vi "Drive.vi"   [LabVIEW 2012]
uses:
  StateMachineType.ctl
  <vilib>/Rock Robotics/WPI/RobotDrive/WPI_RobotDriveGetSetRefNum.vi
  Robot Global Data.vi
types:
  T1 = typedef "StateMachineType.ctl" = enum16{"Init", "Idle", "Start", "Do", "Stop"}
  T2 = typedef "WPI_RobotDriveDevRef.ctl" = cluster{"DevStatus":errorcluster, "Motors[]":T3[], "Square Inputs":bool, "Max Output":dbl, "Isochronous":bool}
  T3 = typedef "WPI_MotorControlDeviceRef.ctl" = cluster{"DeviceStatus":errorcluster, "Type":enum16{"PWM", "CAN"}, "PWM":cluster{"Digital Module":T4, "PWM Channel":T5, "DeadBand":T6}, "CAN":cluster{"Device Number":u8, "Control Mode":T7, "Semaphore":T8, "Max Vout":dbl}, "Invert":bool, "TransformRef":T9, "InvTransformRef":T9}
  T4 = typedef "FPGA_TypedefDigitalModule.ctl" = enum16{"Digital Module 1", "Digital Module 2"}
  T5 = typedef "FPGA_DIOPWMChannel.ctl" = enum8{"PWM 1", "PWM 2", "PWM 3", "PWM 4", "PWM 5", "PWM 6", "PWM 7", "PWM 8", "PWM 9", "PWM 10", "Invalid"}
  T6 = typedef "WPI_PWMDeadband.ctl" = cluster{"Name":string, "maxPositivePwm":i32, "minPositivePwm":i32, "centerPwm":i32, "maxNegativePwm":i32, "minNegativePwm":i32, "angularRange":u16}
  T7 = typedef "WPI_CANJaguar_ControlMode.ctl" = enum8{"Percent VBus", "Current", "Speed", "Position", "Voltage"}
  T8 = typedef "Semaphore RefNum" = refnum<k1>
  T9 = typedef "WPI_PWMTransform_ConPane.ctl" = refnum<vi>
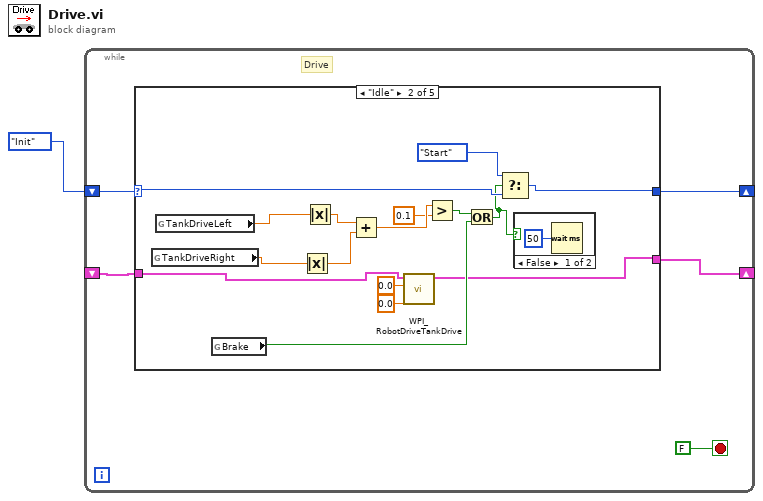
[diagram p0: block diagram]
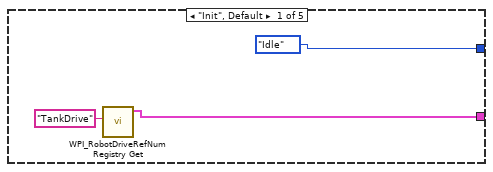
[diagram p2: hidden frame]
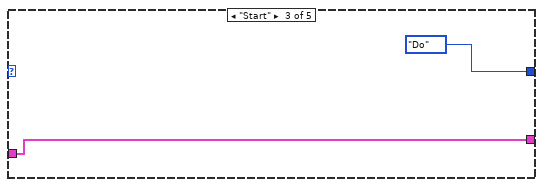
[diagram p4: hidden frame]
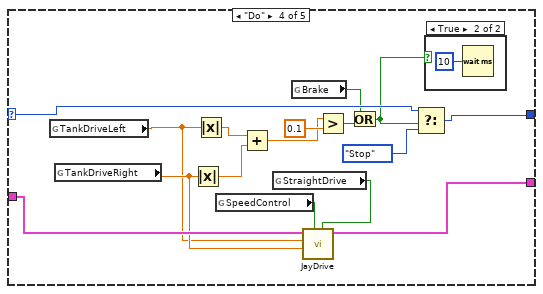
[diagram p5: hidden frame]
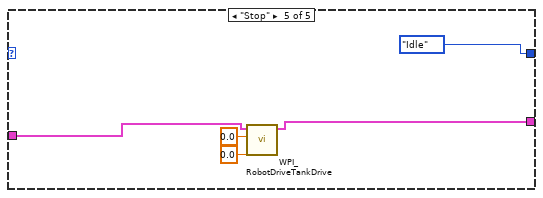
[diagram p7: hidden frame]
diagram:
  n1 = while {
    shift-right: [w4] -> _
    shift-left: StateMachineType."Init" -> [w5]
    shift-right: [w3] -> _
    shift-left: _ -> [w2]
    stop <- FALSE stop-if-true
    # "Drive"
    n2 = case shown="\"Idle\"" w5 {
      selector: w5 -> [_ w20 _ w35 _]
      tunnel: [StateMachineType."Idle" ("Enum") w19 StateMachineType."Do" ("Enum") w36 StateMachineType."Idle" ("Enum")] -> w4
      tunnel: [w7 w10 w28 w37 w48] -> w3
      tunnel: w2 -> [_ w11 w28 w38 w47]
      frame "Init", Default {
        n3 = call <vilib>:"WPI_RobotDriveRefNum Registry Get.vi"("refnum name"="TankDrive") -> ("RobotDriveDevRef"=w7:T2)  [unwired: 9 in, 1 out]
      }
      frame "Idle" {
        n4 = global read "Robot Global Data.vi" "TankDriveRight"() -> (w25:dbl)
        n5 = global read "Robot Global Data.vi" "TankDriveLeft"() -> (w17:dbl)
        n6 = global read "Robot Global Data.vi" "Brake"() -> (w15:bool)
        n7 = Absolute Value(x=w25) -> (abs(x)=w23:dbl)
        n8 = Absolute Value(x=w17) -> (abs(x)=w24:dbl)
        n9 = Add(x=w24, y=w23) -> (x+y=w22:dbl)
        n10 = call <vilib>:"WPI_RobotDriveTankDrive.vi"("Right axis value"=0.0, "Left axis value"=0.0, "RobotDriveDevRef"=w11) -> ("RobotDriveDevRef"=w10:T2)  [unwired: 6 in, 2 out]
        n11 = Greater?(x=w22, y=0.1) -> (0:w16:bool)
        n12 = Or(x=w16, y=w15) -> (x .or. y?=w14:bool)
        n13 = Select(t=StateMachineType."Start" ("Enum"), s=w14, f=w20) -> (s? t:f=w19:T1)
        n14 = case shown="False" w14 {
          frame False {
            n15 = Wait (ms)(milliseconds to wait=u32 50) -> ()  [unwired: 1 out]
          }
          frame True {
          }
        }
      }
      frame "Start" {
      }
      frame "Do" {
        n16 = global read "Robot Global Data.vi" "TankDriveLeft"() -> (w33:dbl)
        n17 = global read "Robot Global Data.vi" "TankDriveRight"() -> (w34:dbl)
        n18 = Absolute Value(x=w34) -> (abs(x)=w40:dbl)
        n19 = Absolute Value(x=w33) -> (abs(x)=w41:dbl)
        n20 = global read "Robot Global Data.vi" "SpeedControl"() -> (w39:bool)
        n21 = Add(x=w41, y=w40) -> (x+y=w43:dbl)
        n22 = global read "Robot Global Data.vi" "StraightDrive"() -> (w32:bool)
        n23 = global read "Robot Global Data.vi" "Brake"() -> (w30:bool)
        n24 = call "JayDrive.vi"("StraightDrive"=w32, "SpeedControl"=w39, "Right Axis"=w34, "Left Axis"=w33, "RobotDriveDevRef"=w38) -> ("RobotDriveDevRef"=w37:T2)  [unwired: 5 in, 1 out]
        n25 = Greater?(x=w43, y=0.1) -> (0:w31:bool)
        n26 = Or(x=w30, y=w31) -> (x .or. y?=w29:bool)
        n27 = Select(t=w35, s=w29, f=StateMachineType."Stop" ("Enum")) -> (s? t:f=w36:T1)
        n28 = case shown="True" w29 {
          frame False {
          }
          frame True {
            n29 = Wait (ms)(milliseconds to wait=u32 10) -> ()  [unwired: 1 out]
          }
        }
      }
      frame "Stop" {
        n30 = call <vilib>:"WPI_RobotDriveTankDrive.vi"("Right axis value"=0.0, "Left axis value"=0.0, "RobotDriveDevRef"=w47) -> ("RobotDriveDevRef"=w48:T2)  [unwired: 6 in, 2 out]
      }
    }
  }
